vi "Do Request.vi"(7 "Processing In":refnum<class "Processing.lvclass">, 11 "Leaderboard in":refnum<class "Leaderboard.lvclass">) -> (0 "error out":errorcluster, 5 "Processing":refnum<class "Processing.lvclass">)   [LabVIEW 2020, in "Summer of LabVIEW.lvlib" / "Leaderboard.lvclass"]
uses:
  Leaderboard.lvclass
  Leaderboard.lvclass/Leaderboard.ctl
  SoL Scoring/Score Entry.ctl
  SoL Scoring/SoL Scoring.lvlib
  SoL Scoring/Score.ctl
  User Score.ctl
  Summer of LabVIEW.lvlib
  Data Types/Challenge JSON.ctl
  Challenge/Challenge.lvclass
  <vilib>/IlluminatedG/lv-web-crypto/lv-json/JSON/JSON.lvlib
  Challenges/Challenges.lvclass
  <vilib>/IlluminatedG/IG HTTP Utils/HTTP Utils/Response/Response.lvclass
  Challenge DB/Challenge DB.lvclass
  <vilib>/IlluminatedG/IG HTTP Server/HTTP Server/Processing/Processing.lvclass
  204d7cf0-41f3-4720-8632-984dbbc5d9e5.vi
  c6e8771d-b672-4ed1-8353-6c6d1ac3a47e.vi
  <vilib>/IlluminatedG/IG HTTP Server/HTTP Server/Security/Security.lvclass
  03a34371-6049-45ae-a150-9db3f9dd66ef.vi
  SQLite/SQLite.lvclass
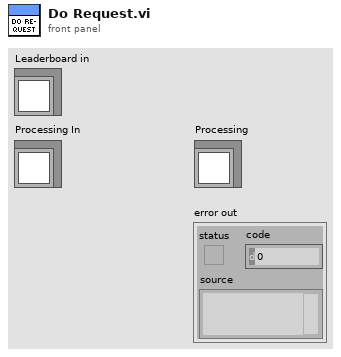
[diagram p1: front panel]
types:
  T1 = typedef "Summer of LabVIEW.lvlib/Challenge JSON.ctl" = cluster{"id":i64, "name":string, "description":string, "download":string, "instructions":string, "start":string, "end":string, "top_subs":T2[]}
  T2 = typedef "Summer of LabVIEW.lvlib/User Score.ctl" = cluster{"first_name":string, "last_name":string, "department":string, "score":T3, "user_id":i64, "sub_id":i64, "chal_id":i64}
  T3 = typedef "SoL Scoring.lvlib/Score.ctl" = cluster{"Overall":dbl, "Categories":T4[]}
  T4 = typedef "SoL Scoring.lvlib/Score Entry.ctl" = cluster{"Category":string, "Value":dbl}
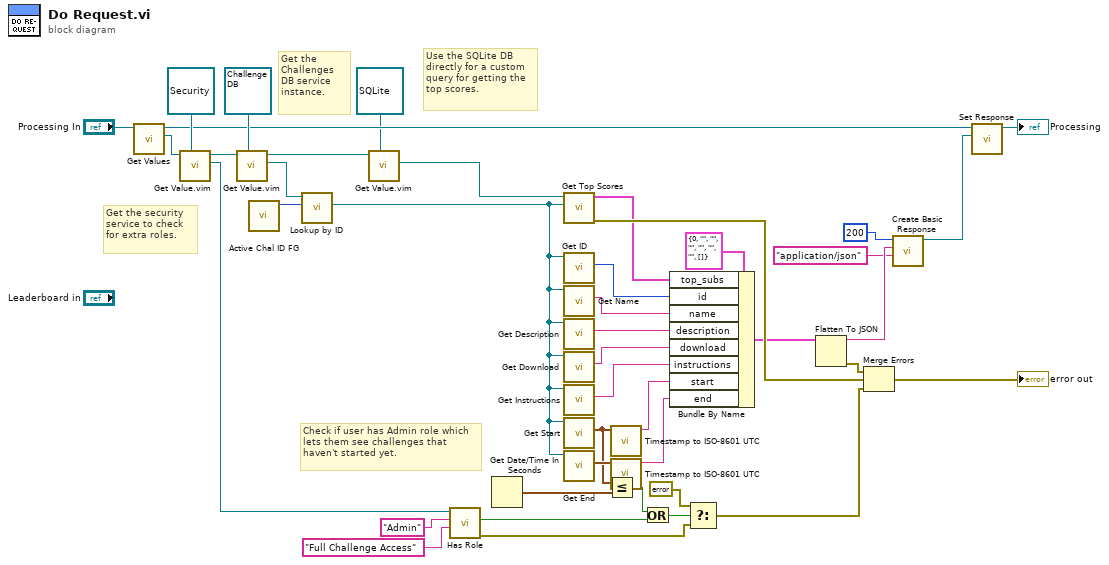
[diagram p0: block diagram]
diagram:
  # "Use the SQLite DB directly for a custom query for getting the top scores."
  # "Get the security service to check for extra roles."
  # "Get the Challenges DB service instance."
  # "Check if user has Admin role which lets them see challenges that haven't started yet."
  n1 = call <vilib>:"Get Values.vi"("Processing in"="Processing In") -> ("Values"=w41:refnum<class "Values.lvclass">, "Processing out"=w34:refnum<class "Processing.lvclass">)  [unwired: 9 in]
  n2 = call "Get Value.vim"("Type / Server / Service (String)"=refnum<class "Security.lvclass"> refnum ("HTTP Server.lvlib:Security.lvclass"), "Arguments in"=w41) -> ("Value"=w39:refnum<class "Security.lvclass">, "Arguments out"=w27:refnum<class "Values.lvclass">)  [unwired: 7 in, 1 out]
  n3 = call "Get Value.vim"("Type / Server / Service (String)"=refnum<class "Challenge DB.lvclass"> refnum ("SOL:Challenge DB.lvclass"), "Arguments in"=w27) -> ("Value"=w7:refnum<class "Challenge DB.lvclass">, "Arguments out"=w33:refnum<class "Values.lvclass">)  [unwired: 7 in, 1 out]
  n4 = call "Active Chal ID FG.vi"() -> ("Active Chal ID"=w6:i64)  [unwired: 11 in]
  n5 = call "Lookup by ID.vi"("ID"=w6, "Challenge DB in"=w7) -> ("Challenge"=w5:refnum<class "Challenge.lvclass">)  [unwired: 6 in, 3 out]
  n6 = call "Get Value.vim"("Type / Server / Service (String)"=refnum<class "SQLite.lvclass"> refnum ("SOL:SQLite"), "Arguments in"=w33) -> ("Value"=w31:refnum<class "SQLite.lvclass">)  [unwired: 7 in, 2 out]
  n7 = call <vilib>:"Has Role.vi"("Description (None)"="Full Challenge Access" ("Role"), "Role"="Admin", "Security in"=w39) -> ("error out"=w3:errorcluster, "Has Role?"=w35:bool)  [unwired: 6 in, 1 out]
  n8 = Get Date/Time In Seconds() -> (seconds since 1Jan1904=w20:timestamp)
  n9 = call "Get Top Scores.vi"("Challenge"=w5, "SQLite"=w31) -> ("error out"=w26:errorcluster, "Top Scores"=w8:T2[])  [unwired: 8 in]
  n10 = call "Get ID.vi"("Challenge in"=w5) -> ("ID"=w16:i64)  [unwired: 9 in, 1 out]
  n11 = call "Get Name.vi"("Challenge in"=w5) -> ("Name"=w17:string)  [unwired: 9 in, 1 out]
  n12 = call "Get Description.vi"("Challenge in"=w5) -> ("Description"=w18:string)  [unwired: 9 in, 1 out]
  n13 = call "Get Download.vi"("Challenge in"=w5) -> ("Download"=w15:string)  [unwired: 9 in, 1 out]
  n14 = call "Get Instructions.vi"("Challenge in"=w5) -> ("Instructions"=w14:string)  [unwired: 9 in, 1 out]
  n15 = call "Get Start.vi"("Challenge in"=w5) -> ("Start"=w10:timestamp)  [unwired: 9 in, 1 out]
  n16 = call "Get End.vi"("Challenge in"=w5) -> ("End"=w13:timestamp)  [unwired: 9 in, 1 out]
  n17 = Less Or Equal?(x=w10, y=w20) -> (x <= y?=w9:bool)
  n18 = call <vilib>:"Timestamp to ISO-8601 UTC.vi"("Time Stamp"=w10) -> ("ISO 8601 UTC"=w12:string)  [unwired: 10 in]
  n19 = call <vilib>:"Timestamp to ISO-8601 UTC.vi"("Time Stamp"=w13) -> ("ISO 8601 UTC"=w11:string)  [unwired: 10 in]
  n20 = Or(x=w9, y=w35) -> (x .or. y?=w4:bool)
  n21 = Bundle By Name(cluster=T1 {"id"=0, "name"="", "description"="", "download"="", "instructions"="", "start"="", "end"="", "top_subs"=[]} ("Challenge JSON"), "top_subs"=w8, "id"=w16, "name"=w17, "description"=w18, "download"=w15, "instructions"=w14, "start"=w12, "end"=w11) -> (w21:T1)
  n22 = Select(t=errorcluster {"status"=FALSE, "code"=0, "source"=""}, s=w4, f=w3) -> (s? t:f=w1:errorcluster)
  n23 = Flatten To JSON(anything=w21) -> (JSON string=w25:string, 11:w22:errorcluster)  [unwired: 2 in]
  n24 = Merge Errors(w22, w26, w1) -> (→"error out":errorcluster)
  n25 = call <vilib>:"Create Basic Response.vi"("Content-Type (text/plain)"="application/json", "Payload"=w25, "Status Code"=u16 200) -> ("Response out"=w36:refnum<class "Response.lvclass">)  [unwired: 7 in, 1 out]
  n26 = call <vilib>:"Set Response.vi"("Response"=w36, "Processing in"=w34) -> ("Processing out"=→"Processing":refnum<class "Processing.lvclass">)  [unwired: 9 in]
